vi "בדיקת צריכת זרם של סליל הפיקוד 5.vi"(7 "resultUserPrompt":bool, 8 "error":errorcluster, 10 "lines":tag="PXI1Slot8/port0/line1", 11 "Path for Log":path) -> (0 "error out":errorcluster, 2 "צריכת זרם בסליל בטווח כן/לא":bool, 3 "צריכת זרם בסליל":dbl format="%.4f")   [LabVIEW 2014]
uses:
  <vilib>/DAQmx/create/channels.llb/DAQmx Create Channel (DO-Digital Output).vi
  <vilib>/DAQmx/write.llb/DAQmx Write (Digital Bool 1Line 1Point).vi
panel:
  # "Right-Click to\nexplain error"
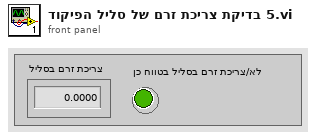
[diagram p1: front panel]
types:
  T1 = enum32{"Invalid", "Standard", "Closed", "Hidden", "Minimized", "Maximized"}
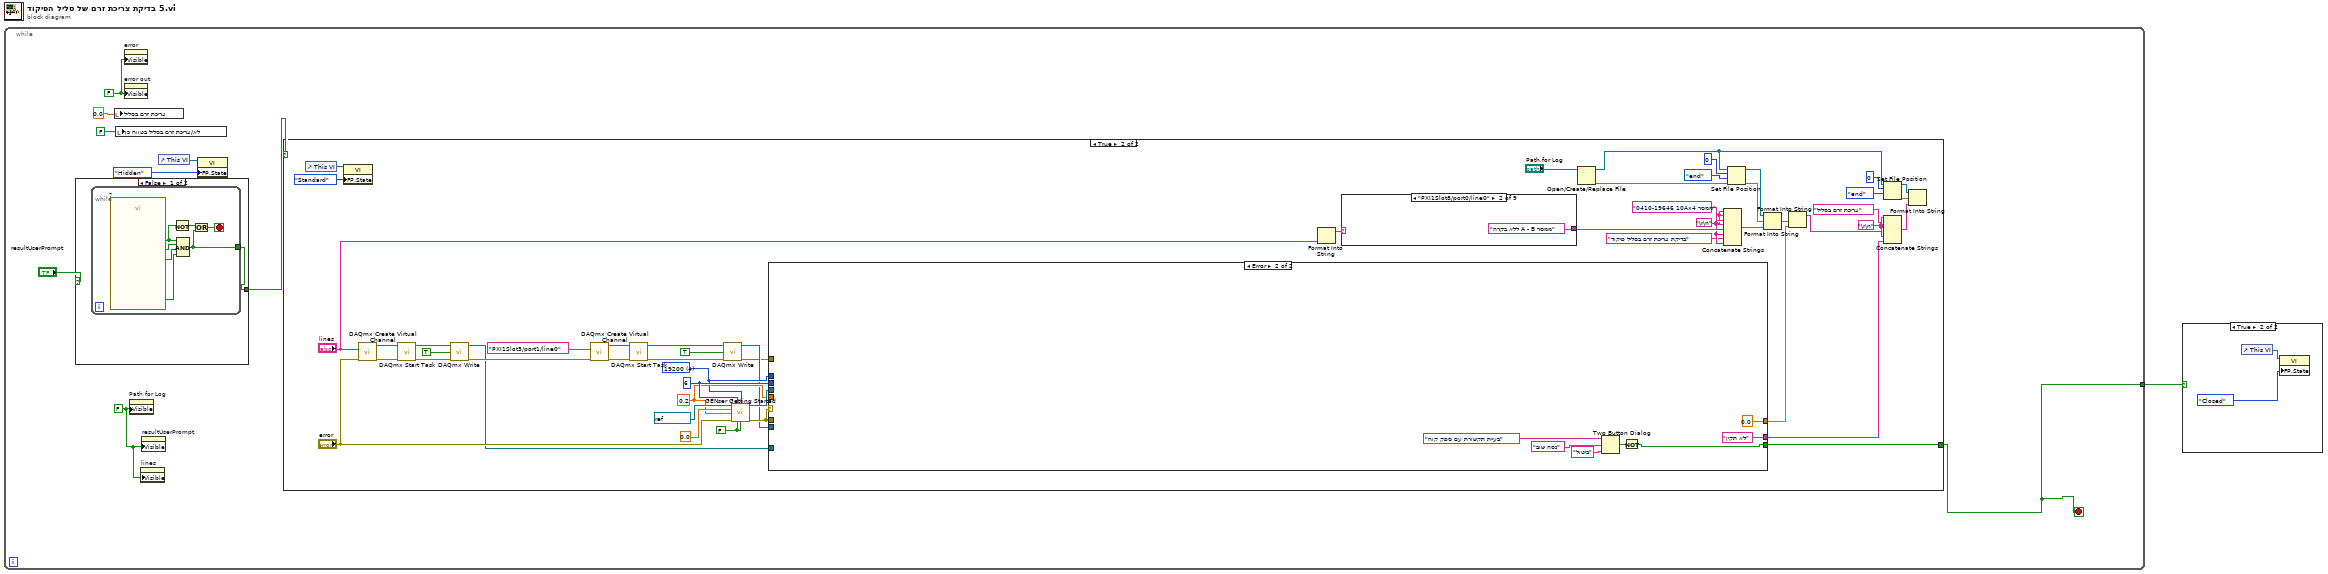
[diagram p0: block diagram]
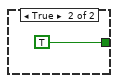
[diagram p3: hidden frame]
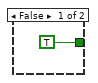
[diagram p4: hidden frame]
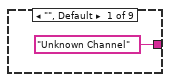
[diagram p5: hidden frame]
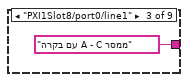
[diagram p6: hidden frame]
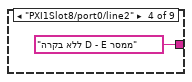
[diagram p7: hidden frame]
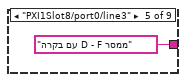
[diagram p8: hidden frame]
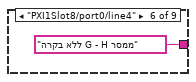
[diagram p9: hidden frame]
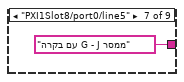
[diagram p10: hidden frame]
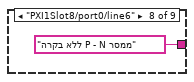
[diagram p11: hidden frame]
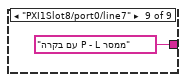
[diagram p12: hidden frame]
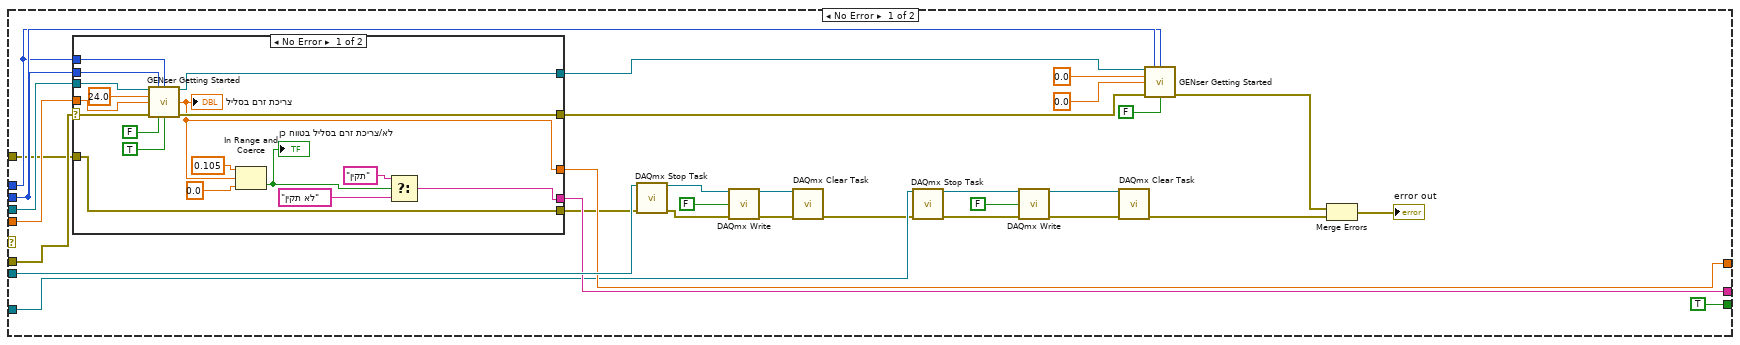
[diagram p13: hidden frame]
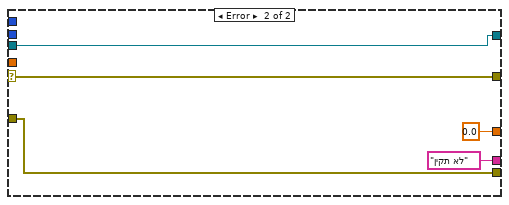
[diagram p14: hidden frame]
diagram:
  n1 = while {
    tunnel: [w2] -> w1
    stop <- w2 stop-if-true
    w3 = FALSE ("Visible")
    w7 = FALSE ("Visible")
    n2 = case shown="False" "resultUserPrompt" {
      tunnel: [w11 TRUE] -> w10
      frame False {
        n3 = while {
          tunnel: [w12] -> w11
          stop <- w14 stop-if-true
          n4 = call "?"() -> ("הדקי הרב מודד"=w16:bool, "M מגע שלילי"=w17:bool, "K מגע חיובי"=w18:bool, "OK"=w13:bool)  [unwired: 15 in, 1 out]
          n5 = Not(x=w13) -> (.not. x?=w15:bool)
          n6 = Compound Arithmetic op=AND(w13, w18, w17, w16) -> (w12:bool)
          n7 = Or(x=w15, y=w12) -> (x .or. y?=w14:bool)
        }
      }
      frame True {
      }
    }
    n8 = local write "צריכת זרם בסליל"(0.0 ("Output Current")) -> ()
    n9 = local write "צריכת זרם בסליל בטווח כן/לא"(FALSE ("In Range?")) -> ()
    n10 = property on="error" class="Clust (strict)"("Visible"=w7) -> ()  [unwired: 2 in, 2 out]
    n11 = property on="error out" class="Clust (strict)"("Visible"=w7) -> ()  [unwired: 2 in, 2 out]
    n12 = property on="Path for Log" class="Path"("Visible"=w3) -> ()  [unwired: 2 in, 2 out]
    n13 = property on="lines" class="DAQmxName"("Visible"=w3) -> ()  [unwired: 2 in, 2 out]
    n14 = property on="resultUserPrompt" class="Bool (strict)"("Visible"=w3) -> ()  [unwired: 2 in, 2 out]
    n15 = control-ref of="This VI"() -> (w6:refnum<vi>)
    n16 = property class="VI"(reference=w6, "FP.State"=T1."Hidden" ("Front Panel Window:State")) -> ()  [unwired: 1 in, 2 out]
    n17 = case shown="True" w10 {
      tunnel: [TRUE ("T button?") w65] -> w2
      frame False {
      }
      frame True {
        w27 = "\r\n"
        w47 = "\r\n"
        w64 = FALSE ("Output On (T)")
        w69 = u16 4 items=["1200", "2400", "4800", "9600", "19200"] ("BAUD")
        w70 = i16 6 ("GEN Addr")
        w66 = 0.2 ("Current Limit")
        n18 = control-ref of="This VI"() -> (w63:refnum<vi>)
        n19 = property class="VI"(reference=w63, "FP.State"=T1."Standard" ("Front Panel Window:State")) -> ()  [unwired: 1 in, 2 out]
        n20 = call-poly <vilib>:"DAQmx Create Virtual Channel.vi"("lines"="lines", "error in"="error") -> ("task out"=w39:refnum<k21>, "error out"=w40:errorcluster)  [unwired: 12 in]
        n21 = call <vilib>:"DAQmx Start Task.vi"("task/channels in"=w39, "error in"=w40) -> ("task out"=w42:refnum<k21>, "error out"=w41:errorcluster)  [unwired: 12 in]
        n22 = call-poly <vilib>:"DAQmx Write.vi"("task/channels in"=w42, "data"=TRUE, "error in"=w41) -> ("task out"=w36:refnum<k21>, "error out"=w37:errorcluster)  [unwired: 10 in, 1 out]
        n23 = call-poly <vilib>:"DAQmx Create Virtual Channel.vi"("lines"=tag "PXI1Slot5/port1/line0", "error in"=w37) -> ("task out"=w60:refnum<k21>, "error out"=w61:errorcluster)  [unwired: 12 in]
        n24 = call <vilib>:"DAQmx Start Task.vi"("task/channels in"=w60, "error in"=w61) -> ("task out"=w58:refnum<k21>, "error out"=w57:errorcluster)  [unwired: 12 in]
        n25 = call-poly <vilib>:"DAQmx Write.vi"("task/channels in"=w58, "data"=TRUE, "error in"=w57) -> ("task out"=w55:refnum<k21>, "error out"=w54:errorcluster)  [unwired: 10 in, 1 out]
        n26 = call "GENser Getting Started.vi"("VISA"=refnum<visa-resource-name> "COM6", "GEN Addr"=w70, "BAUD"=w69, "Voltage Limit"=0.0, "Current Limit"=w66, "error"="error", "Reset (T)"=w64, "Output On (T)"=w64) -> ("VISA out"=w71:refnum<visa-resource-name>, "error out"=w72:errorcluster)  [unwired: 4 in, 2 out]
        n27 = case shown="Error" w72 {
          tunnel: w72 -> [w108 _]
          tunnel: w71 -> [w110 _]
          tunnel: w70 -> [w106 _]
          tunnel: w69 -> [w105 _]
          tunnel: w66 -> [w109 _]
          tunnel: [TRUE w136] -> w65
          tunnel: w55 -> [w104 _]
          tunnel: w54 -> [w100 _]
          tunnel: [w103 0.0 ("Output Current")] -> w53
          tunnel: [w102 "לא תקין"] -> w45
          tunnel: w36 -> [w101 _]
          frame No Error {
            n28 = case shown="No Error" w108 {
              selector: w108 -> [w119 w134]
              tunnel: [w125 w134] -> w111
              tunnel: w105 -> [w124 _]
              tunnel: w106 -> [w123 _]
              tunnel: w110 -> [w122 w135]
              tunnel: w109 -> [w121 _]
              tunnel: [w120 w135] -> w107
              tunnel: [w118 0.0 ("Output Current")] -> w103
              tunnel: [w114 "לא תקין"] -> w102
              tunnel: [w113 w131] -> w99
              tunnel: w100 -> [w113 w131]
              frame No Error {
                n29 = call "GENser Getting Started.vi"("VISA"=w122, "GEN Addr"=w123, "BAUD"=w124, "Voltage Limit"=24.0, "Current Limit"=w121, "error"=w119, "Reset (T)"=FALSE, "Output On (T)"=TRUE) -> ("VISA out"=w120:refnum<visa-resource-name>, "Output Current"=w118:dbl, "error out"=w125:errorcluster)  [unwired: 4 in, 1 out]
                "צריכת זרם בסליל" <- w118
                n30 = In Range and Coerce(upper limit=0.105, x=w118, lower limit=0.0) -> (In Range?=w115:bool)  [unwired: 1 out]
                "צריכת זרם בסליל בטווח כן/לא" <- w115
                n31 = Select(t="תקין", s=w115, f="לא תקין") -> (s? t:f=w114:string)
              }
              frame Error {
              }
            }
            n32 = call <vilib>:"DAQmx Stop Task.vi"("task/channels in"=w104, "error in"=w99) -> ("task out"=w95:refnum<k21>, "error out"=w94:errorcluster)  [unwired: 12 in]
            n33 = call-poly <vilib>:"DAQmx Write.vi"("task/channels in"=w95, "data"=FALSE, "error in"=w94) -> ("task out"=w93:refnum<k21>, "error out"=w92:errorcluster)  [unwired: 10 in, 1 out]
            n34 = call <vilib>:"DAQmx Clear Task.vi"("task in"=w93, "error in"=w92) -> ("error out"=w83:errorcluster)  [unwired: 13 in]
            n35 = call <vilib>:"DAQmx Stop Task.vi"("task/channels in"=w101, "error in"=w83) -> ("task out"=w89:refnum<k21>, "error out"=w87:errorcluster)  [unwired: 12 in]
            n36 = call-poly <vilib>:"DAQmx Write.vi"("task/channels in"=w89, "data"=FALSE, "error in"=w87) -> ("task out"=w86:refnum<k21>, "error out"=w85:errorcluster)  [unwired: 10 in, 1 out]
            n37 = call <vilib>:"DAQmx Clear Task.vi"("task in"=w86, "error in"=w85) -> ("error out"=w84:errorcluster)  [unwired: 13 in]
            n38 = call "GENser Getting Started.vi"("VISA"=w107, "GEN Addr"=w106, "BAUD"=w105, "Voltage Limit"=0.0, "Current Limit"=0.0, "error"=w111, "Output On (T)"=FALSE) -> ("error out"=w82:errorcluster)  [unwired: 5 in, 3 out]
            n39 = Merge Errors(w82, w84) -> (→"error out":errorcluster)
          }
          frame Error {
            n40 = Two Button Dialog(message="בעיית תקשורת עם ספק קוח", 1:"ביטול" ("F button name (\"Cancel\")"), 2:"נסה שוב" ("T button name (\"OK\")")) -> (T button?=w137:bool)
            n41 = Not(x=w137) -> (.not. x?=w136:bool)
          }
        }
        n42 = Format Into String("lines") -> (resulting string=w30:string)  [unwired: 3 in, 1 out]
        n43 = case shown="\"PXI1Slot8/port0/line0\"" w30 {
          tunnel: ["Unknown Channel" "ללא בקרה A - B ממסר" "עם בקרה A - C ממסר" "ללא בקרה D - E ממסר" "עם בקרה D - F ממסר" "ללא בקרה G - H ממסר" "עם בקרה G - J ממסר" "ללא בקרה P - N ממסר" "עם בקרה P - L ממסר"] -> w29
          frame "", Default {
          }
          frame "PXI1Slot8/port0/line0" {
          }
          frame "PXI1Slot8/port0/line1" {
          }
          frame "PXI1Slot8/port0/line2" {
          }
          frame "PXI1Slot8/port0/line3" {
          }
          frame "PXI1Slot8/port0/line4" {
          }
          frame "PXI1Slot8/port0/line5" {
          }
          frame "PXI1Slot8/port0/line6" {
          }
          frame "PXI1Slot8/port0/line7" {
          }
        }
        n44 = Open/Create/Replace File(file path (use dialog)="Path for Log") -> (refnum out=w22:refnum<file>, error out=w33:errorcluster)  [unwired: 5 in, 1 out]
        n45 = Concatenate Strings(w27, w27, "0410-19646 10Ax4 ממסר", w27, w29, w27, "בדיקת צריכת זרם בסליל פיקוד", w27) -> (w32:string)
        n46 = Set File Position(offset (in bytes) (0)=i64 0, refnum=w22, from (0:start)=enum16{"start", "end", "current"}."end", error in=w33) -> (refnum out=w31:refnum<file>, error out=w24:errorcluster)
        n47 = Format Into String(initial string=w31, error in=w24, w32) -> (error out=w23:errorcluster)  [unwired: 1 in, 1 out]
        n48 = Format Into String(error in=w23, w53) -> (resulting string=w44:string)  [unwired: 2 in, 1 out]
        n49 = Set File Position(offset (in bytes) (0)=i64 0, refnum=w22, from (0:start)=enum16{"start", "end", "current"}."end") -> (refnum out=w50:refnum<file>, error out=w51:errorcluster)  [unwired: 1 in]
        n50 = Concatenate Strings(w47, "צריכת זרם בסליל", w47, w44, w47, w45) -> (w52:string)
        n51 = Format Into String(initial string=w50, error in=w51, w52) -> ()  [unwired: 1 in, 2 out]
      }
    }
  }
  n52 = case shown="True" w1 {
    frame False {
    }
    frame True {
      n53 = control-ref of="This VI"() -> (w143:refnum<vi>)
      n54 = property class="VI"(reference=w143, "FP.State"=T1."Closed" ("Front Panel Window:State")) -> ()  [unwired: 1 in, 2 out]
    }
  }
